vi "camera defaults globals.vi"() -> ()   [LabVIEW 2011]
uses:
  image size.ctl
panel:
  in  "Image Size Limits":T1={"Left"=1, "Top"=1, "Right"=2048, "Bottom"=2048, "Binning"=1} {"Binning" items=["1 x 1"=1, "2 x 2"=2, "4 x 4"=4]; "Bottom" min=4 max=2048 step=4; "Right" min=4 max=2048 step=4; "Top" min=1 max=2048 step=4; "Left" min=1 max=2048 step=4}
  in  "Default Image Size":T1={"Left"=1, "Top"=1, "Right"=2048, "Bottom"=2048, "Binning"=1} {"Binning" items=["1 x 1"=1, "2 x 2"=2, "4 x 4"=4]; "Bottom" min=4 max=2048 step=4; "Right" min=4 max=2048 step=4; "Top" min=1 max=2048 step=4; "Left" min=1 max=2048 step=4}
  # "Orca"
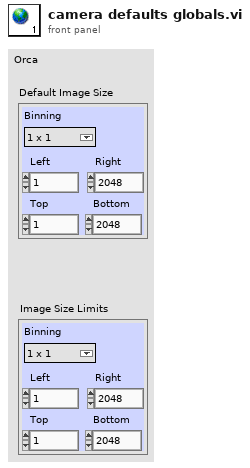
[diagram p1: front panel]
types:
  T1 = typedef "image size.ctl" = cluster{"Left":i32, "Top":i32, "Right":i32, "Bottom":i32, "Binning":u16}
diagram:
